vi "OAT Full Spectrum (2 Ch Even-Angle Signal).vi"(0 "even-angle signals":cluster{"r0":dbl, "dr":dbl, "Y":dbl[]}[](array[cluster]), 1 "even-angle channel info":T9[](array[typedef]) {"channel info"."pregain" format="%.2f"; "channel info"."weighting filter" items=["Linear", "A-weighting", "B-weighting", "C-weighting", "ITU-R 468-4", "Dolby", "CCITT", "C-message", "Wb", "Wc", "Wd", "We", "Wf", "Wh", "Wj", "Wk", "Wm", "AES17 20 kHz lowpass", "AES17 40 kHz lowpass", "AES17 20 kHz highpass", "AES17 40 kHz highpass"]; "channel info"."dB reference" format="%^.1e"; "channel info"."engineering units" items=["custom..."=0, "V"=1, "A"=21, "C"=30, "pC"=31, "s"=32, "-"=29, "Pa"=2, "N"=20, "g"=3, "m/s^2"=4, "m/s"=5, "m"=6, "mm/s"=12, "mm"=13, "micron/s"=14, "micron"=15, "in/s^2"=7, "in/s"=8, "in"=9, "mil/s"=10, "mil"=11, "rad/s^2"=16, "rad/s"=17, "rad"=18, "deg/s^2"=26, "deg/s"=27, "deg"=28, "RPM"=22, "cycle/s^2"=23, "Hz"=24, "cycle"=25, "strain"=19]; "channel info"."sensor sensitivity" format="%#_5f"}, 2 "window (Hanning)":T13=1 items=["None"=0, "Hanning"=1, "Hamming"=2, "Blackman-Harris"=3, "Exact Blackman"=4, "Blackman"=5, "Flat Top"=6, "4 Term B-Harris "=7, "7 Term B-Harris"=8, "Low Sidelobe"=9, "Force - Exponential"=10, "Force"=64, "Exponential"=65, "Blackman Nuttall"=11, "Triangle"=30, "Bartlett-Hanning"=31, "Bohman"=32, "Parzen"=33, "Welch"=34, "Kaiser"=60, "Dolph-Chebyshev"=61, "Gaussian"=62], 3 "block size (-1 = automatic)":i32=-1, 4 "view":T11={"dB On (T)"=FALSE, "unwrap phase (F)"=FALSE, "convert to degree (T)"=TRUE}, 5 "error in (no error)":errorcluster, 6 "rotation direction (CCW)":u16(ring) items=["CCW", "CW"], 7 "averaging parameters":T1={"averaging mode"=enum."No averaging", "weighting mode"=enum."Exponential", "number of averages"=10, "linear mode"=enum."One shot"}, 9 "restart averaging (F)":bool) -> (11 "averaging done":bool, 12 "new spectrum available?":bool, 13 "averages completed":dbl, 14 "full spectrum":T12, 15 "magnitude unit label":string, 16 "phase lag":T8 {"phase" format="%.2f"; "dOrder" format="%.2f"; "Order 0" format="%.2f"}, 17 "phase unit label":string, 18 "spectrum info":T2={"channel name"="", "description"="", "x-axis units"=0, "spectral info"={"spectrum type"=enum."Power [Magnitude^2]", "linear/dB"=enum."linear", "window"=0, "window size"=0, "FFT size"=0}, "engineering units"=0, "custom label"="", "dB reference [EU]"=0.0, "peak units"=enum."rms", "weighting filter"=0, "spectral density?"=FALSE, "unit label"="", "spectrum skewed?"=FALSE, "complimentary spectrum units"=enum."none"} {"x-axis units" items=["Time (s)"=0, "Frequency-CB (Hz)"=1, "Frequency-CPB (Hz)"=1248, "Frequency-Arbitrary (Hz)"=2357, "Quefrency (s)"=2, "Revolutions (rev)"=3, "Order"=4, "Speed (RPM)"=11, "Speed (rad/s)"=21, "Index"=65535]; "weighting filter" items=["Linear", "A-weighting", "B-weighting", "C-weighting", "ITU-R 468-4", "Dolby", "CCITT", "C-message", "Wb", "Wc", "Wd", "We", "Wf", "Wh", "Wj", "Wk", "Wm", "AES17 20 kHz lowpass", "AES17 40 kHz lowpass", "AES17 20 kHz highpass", "AES17 40 kHz highpass"]; "dB reference [EU]" format="%.2f"; "engineering units" items=["custom..."=0, "V"=1, "A"=21, "C"=30, "pC"=31, "s"=32, "-"=29, "Pa"=2, "N"=20, "g"=3, "m/s^2"=4, "m/s"=5, "m"=6, "mm/s"=12, "mm"=13, "micron/s"=14, "micron"=15, "in/s^2"=7, "in/s"=8, "in"=9, "mil/s"=10, "mil"=11, "rad/s^2"=16, "rad/s"=17, "rad"=18, "deg/s^2"=26, "deg/s"=27, "deg"=28, "RPM"=22, "cycle/s^2"=23, "Hz"=24, "cycle"=25, "strain"=19]; "spectral info"."window" items=["None "=0, "Hanning"=1, "Hamming"=2, "Blackman-Harris"=3, "Exact Blackman"=4, "Blackman"=5, "Flat Top"=6, "4 Term B-Harris "=7, "7 Term B-Harris"=8, "Low Sidelobe"=9, "Force - Exponential"=10, "Gaussian"=62]}, 19 "error out":errorcluster)   [LabVIEW 2017, in "SoundVib_OrderTracking.lvlib"]
doc: "This VI computes the full spectrum of a probe pair. The full spectrum provides information on the amplitude of vibration as well as the orbit eccentricity and direction of precession for each frequency/order component."
uses:
  <vilib>/addons/Sound and Vibration/Order Analysis/Resample Order Tracking/SoundVib_OrderTracking.lvlib
  <vilib>/addons/_NISVFA/_Shared subVIs/Controls/svc_Window [Dual FFT].ctl
  <vilib>/addons/_NISVFA/_Shared subVIs/Controls/svc_Resampled Channel Info.ctl
  <vilib>/addons/_NISVFA/_Shared subVIs/Controls/svc_Channel Info.ctl
  <vilib>/addons/_NISVFA/_Shared subVIs/Controls/svc_Engineering Units Text Ring.ctl
  <vilib>/addons/_NISVFA/_Shared subVIs/Controls/svc_Weighting Filter Text Ring.ctl
  <vilib>/addons/_NISVFA/_Shared subVIs/Controls/svc_Spectrum Info.ctl
  <vilib>/addons/_NISVFA/_Shared subVIs/Controls/svc_X-Axis Units.ctl
  <vilib>/addons/_NISVFA/_Shared subVIs/Controls/svc_Spectrum Type.ctl
  <vilib>/addons/_NISVFA/_Shared subVIs/Controls/svc_Complimentary Spectrum Units.ctl
  <vilib>/addons/_NISVFA/_Spectrum Processing/SVFA Unit Conversion (1 Ch).vi
  <vilib>/addons/_NISVFA/_Shared subVIs/Common/svc_Spectrum Units.vi
  <vilib>/addons/_NISVFA/_Spectrum Processing/subVIs/svfa_Conversion Utility (spectrum info).vi
  <vilib>/addons/_NISVFA/_Spectrum Processing/subVIs/svfa_Peak to RMS to Peak2Peak.vi
  <vilib>/addons/_NISVFA/_Spectrum Processing/subVIs/svfa_Mag to Mag2.vi
  <vilib>/addons/_NISVFA/_Spectrum Processing/subVIs/svfa_Linear to dB.vi
  <vilib>/addons/_NISVFA/_Spectrum Processing/subVIs/svfa_dBrefA to dBrefB.vi
  <vilib>/addons/_NISVFA/_Spectrum Processing/subVIs/svfa_Spectrum to Spectral Density.vi
  <vilib>/addons/_NISVFA/_Shared subVIs/Common/svc_Get Weighting Enum and Labels.vi
  <vilib>/addons/_NISVFA/_Shared subVIs/Common/svc_Unit Label Lexical Class.vi
  <vilib>/addons/_NISVFA/_Shared subVIs/Common/svc_Engineering Units to Unit Label.vi
  <vilib>/addons/_NISVFA/_Shared subVIs/Common/svc_Format Value (DBL).vi
  <vilib>/addons/_NISVFA/_Shared subVIs/Common/svc_Window Parameters.vi
  <vilib>/addons/_NISVFA/_Spectrum Processing/SVFA Wrap or Unwrap Phase (1 Ch).vi
  <vilib>/addons/_NISVFA/_Spectrum Processing/SVFA Phase Unit Conversion (1 Ch).vi
  <vilib>/addons/_NISVFA/_Spectrum Processing/SVFA Unit Conversion (N Ch).vi
  <vilib>/addons/Sound and Vibration/Order Analysis/Resample Order Tracking/OAT Order Power Spectrum (N Channels).vi
  <vilib>/addons/Sound and Vibration/Order Analysis/Utility/OAT Output Triggered Even Angle Signal (N Channels).vi
  <vilib>/addons/Sound and Vibration/Order Analysis/Utility/SoundVib_OAUtility.lvlib
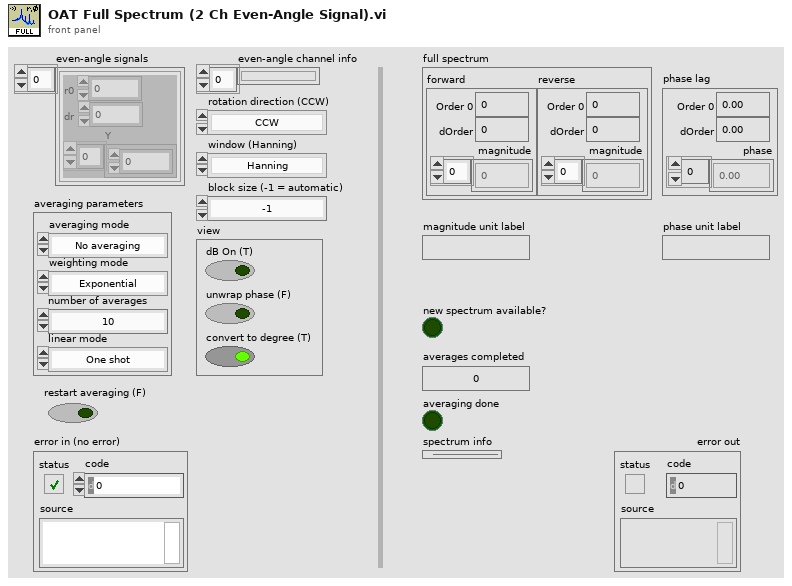
[diagram p1: front panel]
types:
  T1 = cluster{"averaging mode":enum16{"No averaging", "Vector averaging", "RMS averaging", "Peak hold"}, "weighting mode":enum16{"Linear", "Exponential"}, "number of averages":u32, "linear mode":enum16{"One shot", "Auto restart"}}
  T2 = typedef "svc_Spectrum Info.ctl" = cluster{"channel name":string, "description":string, "x-axis units":T3, "spectral info":cluster{"spectrum type":T4, "linear/dB":enum16{"linear", "dB"}, "window":u16, "window size":i32, "FFT size":i32}, "engineering units":T5, "custom label":string, "dB reference [EU]":dbl, "peak units":enum16{"rms", "peak", "peak-peak"}, "weighting filter":T6, "spectral density?":bool, "unit label":string, "spectrum skewed?":bool, "complimentary spectrum units":T7}
  T3 = typedef "svc_X-Axis Units.ctl" = u16
  T4 = typedef "svc_Spectrum Type.ctl" = enum16{"FFT Spectrum [complex]", "Amplitude [Magnitude]", "Power [Magnitude^2]", "Cross Spectrum [complex]", "Frequency Response [Complex]"}
  T5 = typedef "svc_Engineering Units Text Ring.ctl" = u16
  T6 = typedef "svc_Weighting Filter Text Ring.ctl" = u16
  T7 = typedef "svc_Complimentary Spectrum Units.ctl" = enum16{"none", "radians", "degrees", "cycles", "imaginary"}
  T8 = cluster{"Order 0":dbl, "dOrder":dbl, "phase":dbl[]}
  T9 = typedef "svc_Resampled Channel Info.ctl" = cluster{"channel name":string, "description":string, " channel info":T10}
  T10 = typedef "svc_Channel Info.ctl" = cluster{"sensor sensitivity":dbl, "engineering units":T5, "dB reference":dbl, "custom label":string, "weighting filter":T6, "pregain":dbl}
  T11 = cluster{"dB On (T)":bool, "unwrap phase (F)":bool, "convert to degree (T)":bool}
  T12 = cluster{"forward":cluster{"Order 0":dbl, "dOrder":dbl, "magnitude":dbl[]}, "reverse":cluster{"Order 0":dbl, "dOrder":dbl, "magnitude":dbl[]}}
  T13 = typedef "svc_Window [Dual FFT].ctl" = u32
  T14 = cluster{"linear/dB":enum16{"no change", "linear", "dB"}, "dB reference (0: no change)":dbl, "power/magnitude":enum16{"no change", "power", "magnitude"}, "view":enum16{"no change", "rms", "peak", "peak-peak"}}
  T15 = enum16{"No change", "Radians", "Degrees", "Cycles"}
  T16 = enum16{"No change", "Unwrap", "Wrap: -360 to 0", "Wrap: -270 to 90", "Wrap: -180 to 180", "Wrap: -90 to 270", "Wrap: 0 to 360", "Wrap: custom range"}
  T17 = cluster{"forward":cluster{"x0":dbl, "dx":dbl, "magnitude":dbl[]}, "reverse":cluster{"x0":dbl, "dx":dbl, "magnitude":dbl[]}}
  T18 = enum16{"No averaging", "Vector averaging", "RMS averaging", "Peak hold"}
  T19 = cluster{"order 0":dbl, "delta order":dbl, "magnitude":dbl[]}[]
  T20 = cluster{"order 0":dbl, "delta order":dbl, "magnitude":dbl[]}
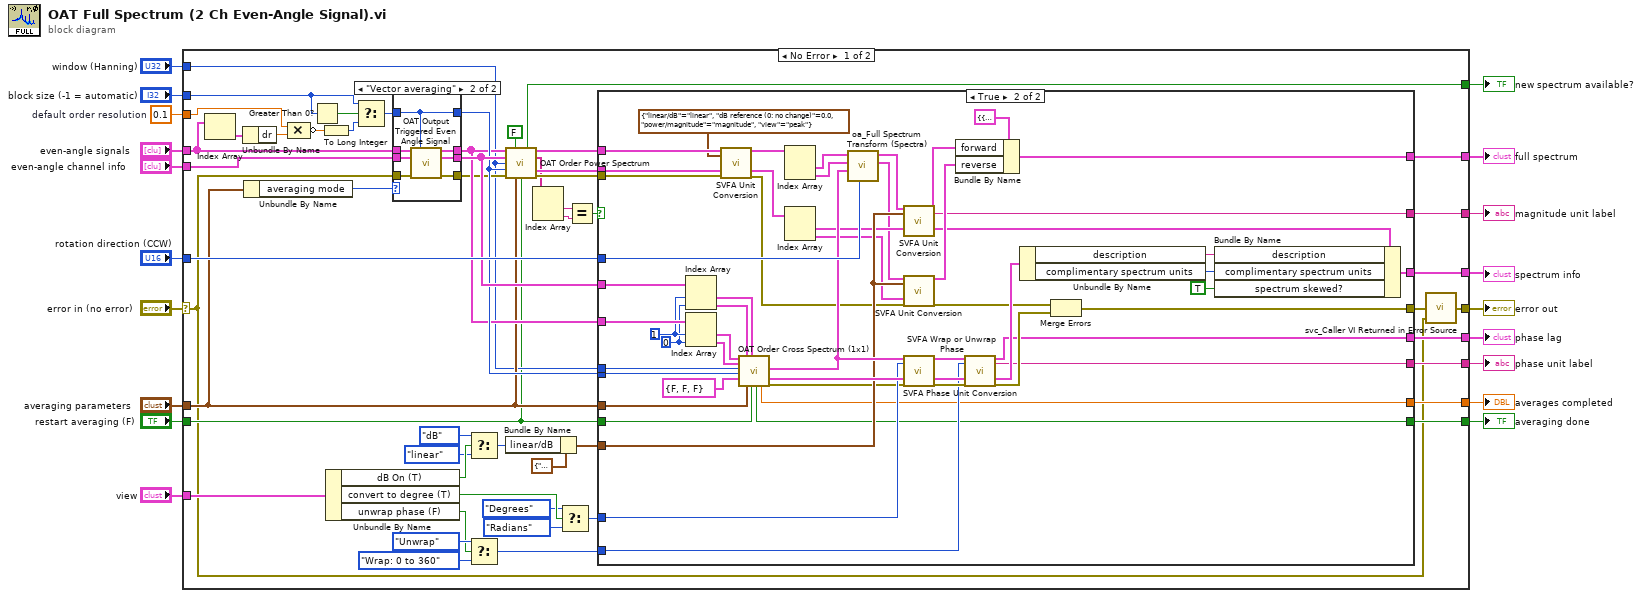
[diagram p0: block diagram]
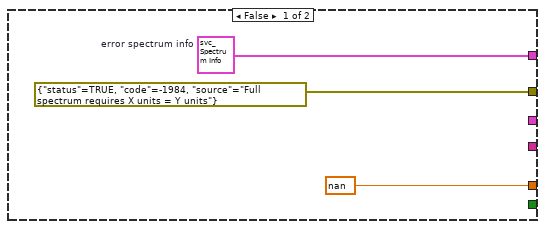
[diagram p2: hidden frame]
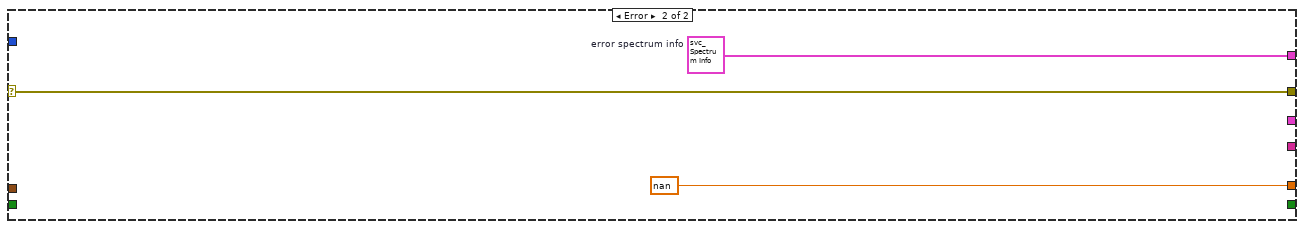
[diagram p4: hidden frame]
diagram:
  w2 = 0.1  # default order resolution
  n1 = case shown="No Error" "error in (no error)" {
    selector: "error in (no error)" -> [w35 w142]
    tunnel: "rotation direction (CCW)" -> [w72 _]
    tunnel: [w70 _] -> w18
    tunnel: "even-angle signals" -> [w29 _]
    tunnel: "averaging parameters" -> [w62 _]
    tunnel: "view" -> [w50 _]
    tunnel: [w46 nan ("averages completed")] -> w14
    tunnel: [w45 _] -> w13
    tunnel: [w34 w142] -> w12
    tunnel: [w43 _] -> w11
    tunnel: [w42 _] -> w10
    tunnel: [w41 _] -> w9
    tunnel: [w40 w141] -> w8
    tunnel: "block size (-1 = automatic)" -> [w21 _]
    tunnel: "window (Hanning)" -> [w39 _]
    tunnel: "even-angle channel info" -> [w38 _]
    tunnel: "restart averaging (F)" -> [w37 _]
    tunnel: w2 -> [w22 _]
    tunnel: [w20 _] -> w1
    frame No Error {
      n2 = Index Array(array=w29) -> (element=w28:cluster{"r0":dbl, "dr":dbl, "Y":dbl[]})  [unwired: 1 in]
      n3 = Unbundle By Name(w28) -> ("dr"=w27:dbl)
      n4 = Unbundle By Name(w62) -> ("averaging mode"=w63:T18)
      n5 = Compound Arithmetic op=MULTIPLY(w22, w27) -> (invert w26:dbl)
      n6 = Greater Than 0?(x=w21) -> (x > 0?=w25:bool)
      n7 = To Long Integer(number=w26) -> (32bit integer=w24:i32)
      n8 = Unbundle By Name(w50) -> ("dB On (T)"=w60:bool, "convert to degree (T)"=w56:bool, "unwrap phase (F)"=w51:bool)
      n9 = Select(t=w21, s=w25, f=w24) -> (s? t:f=w23:i32)
      n10 = case shown="\"Vector averaging\"" w63 {
        tunnel: w35 -> [w132 w140]
        tunnel: [w132 w139] -> w64
        tunnel: w23 -> [w133 w134]
        tunnel: [w133 w134] -> w67
        tunnel: w29 -> [w130 w138]
        tunnel: w38 -> [w131 w137]
        tunnel: [w131 w135] -> w71
        tunnel: [w130 w136] -> w66
        frame "No averaging", Default {
        }
        frame "Vector averaging" {
          n11 = call-poly <vilib>:"OAT Output Triggered Even Angle Signal.vi"("even-angle signals"=w138, "block size"=w134, "even-angle channel info"=w137, "error in (no error)"=w140) -> ("triggered even-angle signals"=w136:cluster{"r0":dbl, "dr":dbl, "Y":dbl[]}[], "even-angle channel info out"=w135:T9[], "error out"=w139:errorcluster)  [unwired: 9 in]
        }
      }
      n12 = Select(t=enum16{"no change", "linear", "dB"}."dB" ("linear/dB"), s=w60, f=enum16{"no change", "linear", "dB"}."linear" ("linear/dB")) -> (s? t:f=w61:enum16{"no change", "linear", "dB"})
      n13 = Select(t=T16."Unwrap" ("desired wrapping"), s=w51, f=T16."Wrap: 0 to 360" ("desired wrapping")) -> (s? t:f=w48:T16)
      n14 = call-poly <vilib>:"OAT Order Power Spectrum.vi"("even-angle signals"=w66, "dB on? (T)"=FALSE, "even-angle channel info"=w71, "window"=w39, "block size"=w67, "error in (no error)"=w64, "averaging parameters"=w62, "restart averaging? (F)"=w37) -> ("new spectrum available?"=w20:bool, "order power spectra"=w68:T19, "unit labels"=w32:string[], "spectrum info"=w69:T2[], "error out"=w44:errorcluster)  [unwired: 1 in, 2 out]
      n15 = Bundle By Name(cluster=T14 {"linear/dB"=enum."no change", "dB reference (0: no change)"=0.0, "power/magnitude"=enum."no change", "view"=enum."no change"} ("desired scaling"), "linear/dB"=w61) -> (w47:T14)
      n16 = Index Array(array=w32) -> (element #1=w31:string, element #2=w30:string)  [unwired: 2 in]
      n17 = Select(t=T15."Degrees" ("desired units"), s=w56, f=T15."Radians" ("desired units")) -> (s? t:f=w49:T15)
      n18 = Equal?(x=w31, y=w30) -> (x = y?=w36:bool)
      n19 = case shown="True" w36 {
        tunnel: w72 -> [_ w128]
        tunnel: w71 -> [_ w125]
        tunnel: [_ w124] -> w70
        tunnel: w69 -> [_ w120]
        tunnel: w68 -> [_ w119]
        tunnel: w67 -> [_ w118]
        tunnel: w66 -> [_ w117]
        tunnel: w62 -> [_ w116]
        tunnel: w49 -> [_ w109]
        tunnel: w48 -> [_ w108]
        tunnel: w47 -> [_ w107]
        tunnel: [nan ("averages completed") w99] -> w46
        tunnel: [_ w98] -> w45
        tunnel: w44 -> [_ w91]
        tunnel: [errorcluster {"status"=TRUE, "code"=-1984, "source"="Full spectrum requires X units = Y units"} ("error IO") w88] -> w33
        tunnel: [_ w87] -> w43
        tunnel: [_ w86] -> w42
        tunnel: [_ w85] -> w41
        tunnel: [w73 w83] -> w40
        tunnel: w39 -> [_ w82]
        tunnel: w37 -> [_ w77]
        frame False {
          w73 = T2 {"channel name"="Error", "description"="Error", "x-axis units"=99, "spectral info"={"spectrum type"=enum."Power [Magnitude^2]", "linear/dB"=enum."linear", "window"=99, "window size"=-1, "FFT size"=-1}, "engineering units"=0, "custom label"="Error", "dB reference [EU]"=0.0, "peak units"=enum."rms", "weighting filter"=0, "spectral density?"=FALSE, "unit label"="Error", "spectrum skewed?"=FALSE, "complimentary spectrum units"=enum."none"}  # error spectrum info
        }
        frame True {
          w78 = 0 ("index")
          w79 = 1 ("index")
          n20 = Index Array(array=w125, index #1=w79, index #2=w78) -> (element #1=w126:T9, element #2=w127:T9)
          n21 = Index Array(array=w117, index #1=w79, index #2=w78) -> (element #1=w80:cluster{"r0":dbl, "dr":dbl, "Y":dbl[]}, element #2=w81:cluster{"r0":dbl, "dr":dbl, "Y":dbl[]})
          n22 = call-poly <vilib>:"SVFA Unit Conversion.vi"("spectra"=w119, "desired scaling"=T14 {"linear/dB"=enum."linear", "dB reference (0: no change)"=0.0, "power/magnitude"=enum."magnitude", "view"=enum."peak"}, "spectrum info in"=w120, "error in (no error)"=w91) -> ("converted spectra"=w121:cluster{"x0":dbl, "dx":dbl, "magnitude":dbl[]}[], "spectrum info out"=w105:T2[], "error out"=w90:errorcluster)  [unwired: 12 in, 1 out]
          n23 = call <vilib>:"OAT Order Cross Spectrum (1x1).vi"("even-angle signal X"=w80, "even-angle signal Y"=w81, "window"=w82, "block size"=w118, "view"=T11 {"dB On (T)"=FALSE, "unwrap phase (F)"=FALSE, "convert to degree (T)"=FALSE}, "even-angle channel info X"=w127, "averaging parameters"=w116, "even-angle channel info Y"=w126, "restart averaging? (F)"=w77) -> ("averaging done?"=w98:bool, "averages completed"=w99:dbl, "cross spectrum phase"=w111:T20, "spectrum info"=w110:T2, "error out"=w92:errorcluster)  [unwired: 2 in, 4 out]
          n24 = Index Array(array=w121) -> (element #1=w122:cluster{"x0":dbl, "dx":dbl, "magnitude":dbl[]}, element #2=w123:cluster{"x0":dbl, "dx":dbl, "magnitude":dbl[]})  [unwired: 2 in]
          n25 = Index Array(array=w105) -> (element #1=w104:T2, element #2=w102:T2)  [unwired: 2 in]
          n26 = call <vilib>:"oa_Full Spectrum Transform (Spectra).vi"("direction"=w128, "phase lag spectrum (X-Y)"=w111, "Y magnitude spectrum"=w123, "X magnitude spectrum"=w122) -> ("reverse precession spectrum"=w103:cluster{"x0":dbl, "dx":dbl, "magnitude":dbl[]}, "forward precession spectrum"=w106:cluster{"x0":dbl, "dx":dbl, "magnitude":dbl[]})  [unwired: 6 in]
          n27 = call-poly <vilib>:"SVFA Unit Conversion.vi"("spectrum"=w106, "desired scaling"=w107, "spectrum info in"=w104) -> ("converted spectrum"=w101:cluster{"x0":dbl, "dx":dbl, "magnitude":dbl[]}, "unit label"=w87:string, "spectrum info out"=w84:T2)  [unwired: 13 in, 1 out]
          n28 = call-poly <vilib>:"SVFA Unit Conversion.vi"("spectrum"=w103, "desired scaling"=w107, "spectrum info in"=w102, "error in (no error)"=w90) -> ("converted spectrum"=w100:cluster{"x0":dbl, "dx":dbl, "magnitude":dbl[]}, "error out"=w89:errorcluster)  [unwired: 12 in, 2 out]
          n29 = call-poly <vilib>:"SVFA Phase Unit Conversion.vi"("phase spectrum"=w111, "desired units"=w109, "spectrum info in"=w110, "error in (no error)"=w92) -> ("converted phase spectrum"=w112:cluster{"f0":dbl, "df":dbl, "phase":dbl[]}, "spectrum info out"=w113:T2, "error out"=w114:errorcluster)  [unwired: 12 in, 1 out]
          n30 = Bundle By Name(cluster=T17 {"forward"={"x0"=0.0, "dx"=0.0, "magnitude"=[]}, "reverse"={"x0"=0.0, "dx"=0.0, "magnitude"=[]}}, "forward"=w101, "reverse"=w100) -> (w124:T17)
          n31 = call-poly <vilib>:"SVFA Wrap or Unwrap Phase.vi"("phase spectrum in"=w112, "desired wrapping"=w108, "spectrum info"=w113, "error in (no error)"=w114) -> ("phase spectrum out"=w86:cluster{"f0":dbl, "df":dbl, "phase":dbl[]}, "unit label"=w85:string, "dup spectrum info"=w94:T2, "error out"=w93:errorcluster)  [unwired: 12 in]
          n32 = Unbundle By Name(w94) -> ("description"=w95:string, "complimentary spectrum units"=w96:T7)
          n33 = Merge Errors(w89, w93) -> (w88:errorcluster)
          n34 = Bundle By Name(cluster=w84, "description"=w95, "complimentary spectrum units"=w96, "spectrum skewed?"=TRUE) -> (w83:T2)
        }
      }
      n35 = call <vilib>:"svc_Caller VI Returned in Error Source.vi"("warning input to caller"=w35, "error in (no error)"=w33) -> ("error out"=w34:errorcluster)  [unwired: 3 in]
    }
    frame Error {
      w141 = T2 {"channel name"="Error", "description"="Error", "x-axis units"=99, "spectral info"={"spectrum type"=enum."Power [Magnitude^2]", "linear/dB"=enum."linear", "window"=99, "window size"=-1, "FFT size"=-1}, "engineering units"=0, "custom label"="Error", "dB reference [EU]"=0.0, "peak units"=enum."rms", "weighting filter"=0, "spectral density?"=FALSE, "unit label"="Error", "spectrum skewed?"=FALSE, "complimentary spectrum units"=enum."none"}  # error spectrum info
    }
  }
  "full spectrum" <- w18
  "phase lag" <- w10
  "error out" <- w12
  "magnitude unit label" <- w11
  "phase unit label" <- w9
  "averages completed" <- w14
  "averaging done" <- w13
  "spectrum info" <- w8
  "new spectrum available?" <- w1
